vi "Manage Setpoint Channel.vi"(8 "error in (no error)":errorcluster, 10 "Use External Setpoint":bool, 11 "Node Ptr":T1 format="%.0x") -> (0 "error out":errorcluster, 3 "Node Ptr out":T1 format="%.0x")   [LabVIEW 2013, in "Control Addon System Explorer.lvlib"]
uses:
  Control Addon System Explorer.lvlib
  <vilib>/NI Veristand/Custom Device API/Custom Device Item Ref.ctl
  <vilib>/NI Veristand/Custom Device API/Custom Device Channel.ctl
  <vilib>/NI Veristand/Custom Device API/Custom Device Channel Type.ctl
  Shared/Constants.vi
  <vilib>/NI Veristand/Custom Device Tools/Custom Device Utility Library/NI VeriStand - Search for Item by GUID.vi
  Shared/Control Addon Shared.lvlib
  <vilib>/NI Veristand/Custom Device API/Custom Device API.lvlib
  <vilib>/NI Veristand/Custom Device Tools/Custom Device Utility Library/Custom Device Utility Library.lvlib
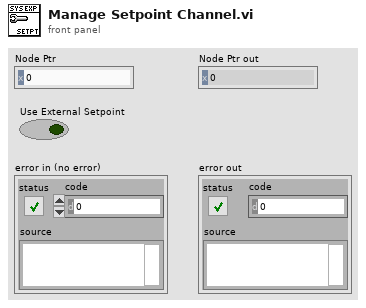
[diagram p1: front panel]
types:
  T1 = typedef "Custom Device API.lvlib/Custom Device Item Ref.ctl" = u64
  T2 = typedef "Custom Device API.lvlib/Custom Device Channel.ctl" = cluster{"Type":T3, "Units":string, "Default Value":dbl, "Faultable":bool, "Scalable":bool}
  T3 = typedef "Custom Device API.lvlib/Custom Device Channel Type.ctl" = enum16{"Input", "Output"}
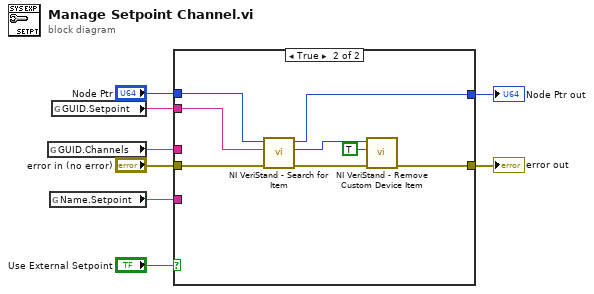
[diagram p0: block diagram]
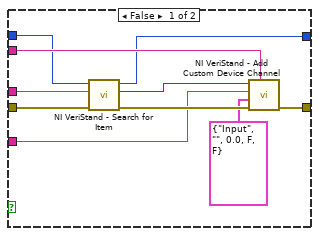
[diagram p2: hidden frame]
diagram:
  n1 = global read "Constants.vi" "GUID.Channels"() -> (w2:string)
  n2 = global read "Constants.vi" "Name.Setpoint"() -> (w3:string)
  n3 = global read "Constants.vi" "GUID.Setpoint"() -> (w1:string)
  n4 = case shown="True" "Use External Setpoint" {
    tunnel: w1 -> [w14 w26]
    tunnel: w2 -> [w16 _]
    tunnel: w3 -> [w13 _]
    tunnel: [w12 w21] -> w4
    tunnel: "error in (no error)" -> [w11 w25]
    tunnel: "Node Ptr" -> [w10 w20]
    tunnel: [w9 w19] -> w7
    frame False {
      n5 = call-poly <vilib>:"NI VeriStand - Search for Item.vi"("error in"=w11, "Item GUID"=w16, "Section Ref in"=w10) -> ("error out"=w18:errorcluster, "Item Ref"=w17:T1, "Section Ref out"=w9:T1)  [unwired: 5 in, 1 out]
      n6 = call <vilib>:"NI VeriStand - Add Custom Device Channel.vi"("GUID (Default Channel)"=w14, "error in (no error)"=w18, "Channel"=T2 {"Type"=enum."Input", "Units"="", "Default Value"=0.0, "Faultable"=FALSE, "Scalable"=FALSE}, "Channel Name"=w13, "Parent Ref in"=w17) -> ("error out"=w12:errorcluster)  [unwired: 3 in, 3 out]
    }
    frame True {
      n7 = call-poly <vilib>:"NI VeriStand - Search for Item.vi"("error in"=w25, "Item GUID"=w26, "Section Ref in"=w20) -> ("error out"=w24:errorcluster, "Item Ref"=w23:T1, "Section Ref out"=w19:T1)  [unwired: 5 in, 1 out]
      n8 = call <vilib>:"NI VeriStand - Remove Custom Device Item.vi"("error in (no error)"=w24, "Force Delete (F)"=TRUE, "Item Ref in"=w23) -> ("error out"=w21:errorcluster)  [unwired: 7 in, 1 out]
    }
  }
  "Node Ptr out" <- w7
  "error out" <- w4
